vi "dsdll_signal_demo.vi"() -> ()   [LabVIEW 2020, in "dsdll.lvlib"]
doc: "Simple DSDLL demo for measurement of two port system amplitude and phase transfer. \n\nIt generates white noise on mono output and periodically captures waveforms at stereo inputs. \nCaptured wavefroms are displayed and their spectra are calculated. Ratio of their spectra (system frequency response) is filtered and displayed in frequency domain and in nyquist plot."
uses:
  dsdll.lvlib
  dsdll_instance.ctl
  dsdll_device_record.ctl
  dsdll_format.ctl
  dsdll_sample_format.ctl
  dsdll_capture_wave_auto_float32.vi
  dsdll_output_write_auto_float32.vi
panel:
  in  "cut freq":dbl=20000.0 caption="Cut off frequency [Hz]" format="%#_6p"
  out "Nyquist":cluster{dbl[], dbl[]}(graph)
  in  "capt n":u16(ring)=512 caption="Capture samples" items=["64"=64, "128"=128, "256"=256, "512"=512, "1024"=1024, "2048"=2048, "4096"=4096]
  in  "srate":u32=48000 caption="Sample rate [Hz]"
  out "Waveforms":cluster{"fscale":dbl[], dbl[]}[](graph)
  out "A":cdb[](array[numeric])
  out "Transfer":cluster{"fscale":dbl[], dbl[]}[](graph)
  in  "refresh":i32=10 caption="Refresh [ms]" min=0
  in  "btn clr avg":bool
  in  "avg n":u32=5 caption="Averages" min=1
  in  "gen N":i32=7919 caption="Noise generator period"
  in  "btn close":bool
  in  "btn open":bool
  in  "btn exit":bool
  in  "devs capt":u16(ring) caption="Capture devices"
  in  "devs out":u16(ring) caption="Output devices"
  in  "btn enum":bool
  out "error out":errorcluster caption="Error out"
  out "dsdll":T1
  # "DSDLL: Frequency response demo"
  # "Sound card connection:"
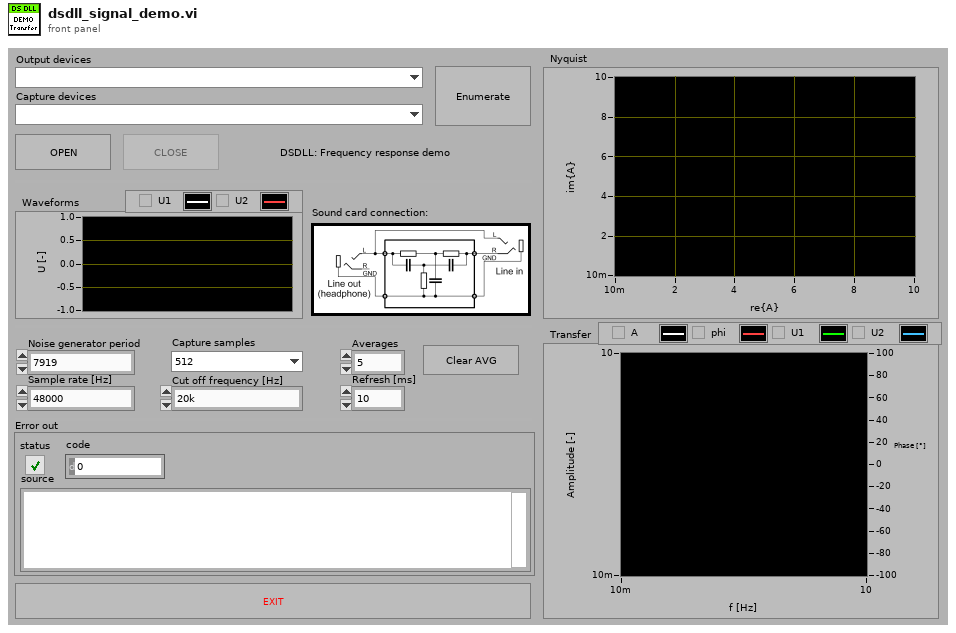
[diagram p1: front panel]
types:
  T1 = typedef "dsdll.lvlib/dsdll_instance.ctl" = cluster{"dsdll path":path, "dsdll handle":u8[], "output devices":T2[], "capture devices":T2[]}
  T2 = typedef "dsdll.lvlib/dsdll_device_record.ctl" = cluster{"guid":u8[], "name":string}
  T3 = typedef "dsdll.lvlib/dsdll_format.ctl" = cluster{"sample rate [Hz]":u32, "out channels":u16, "inp channels":u16, "format":T4}
  T4 = typedef "dsdll.lvlib/dsdll_sample_format.ctl" = enum16{"IEEE float 32", "PCM 16 bit"}
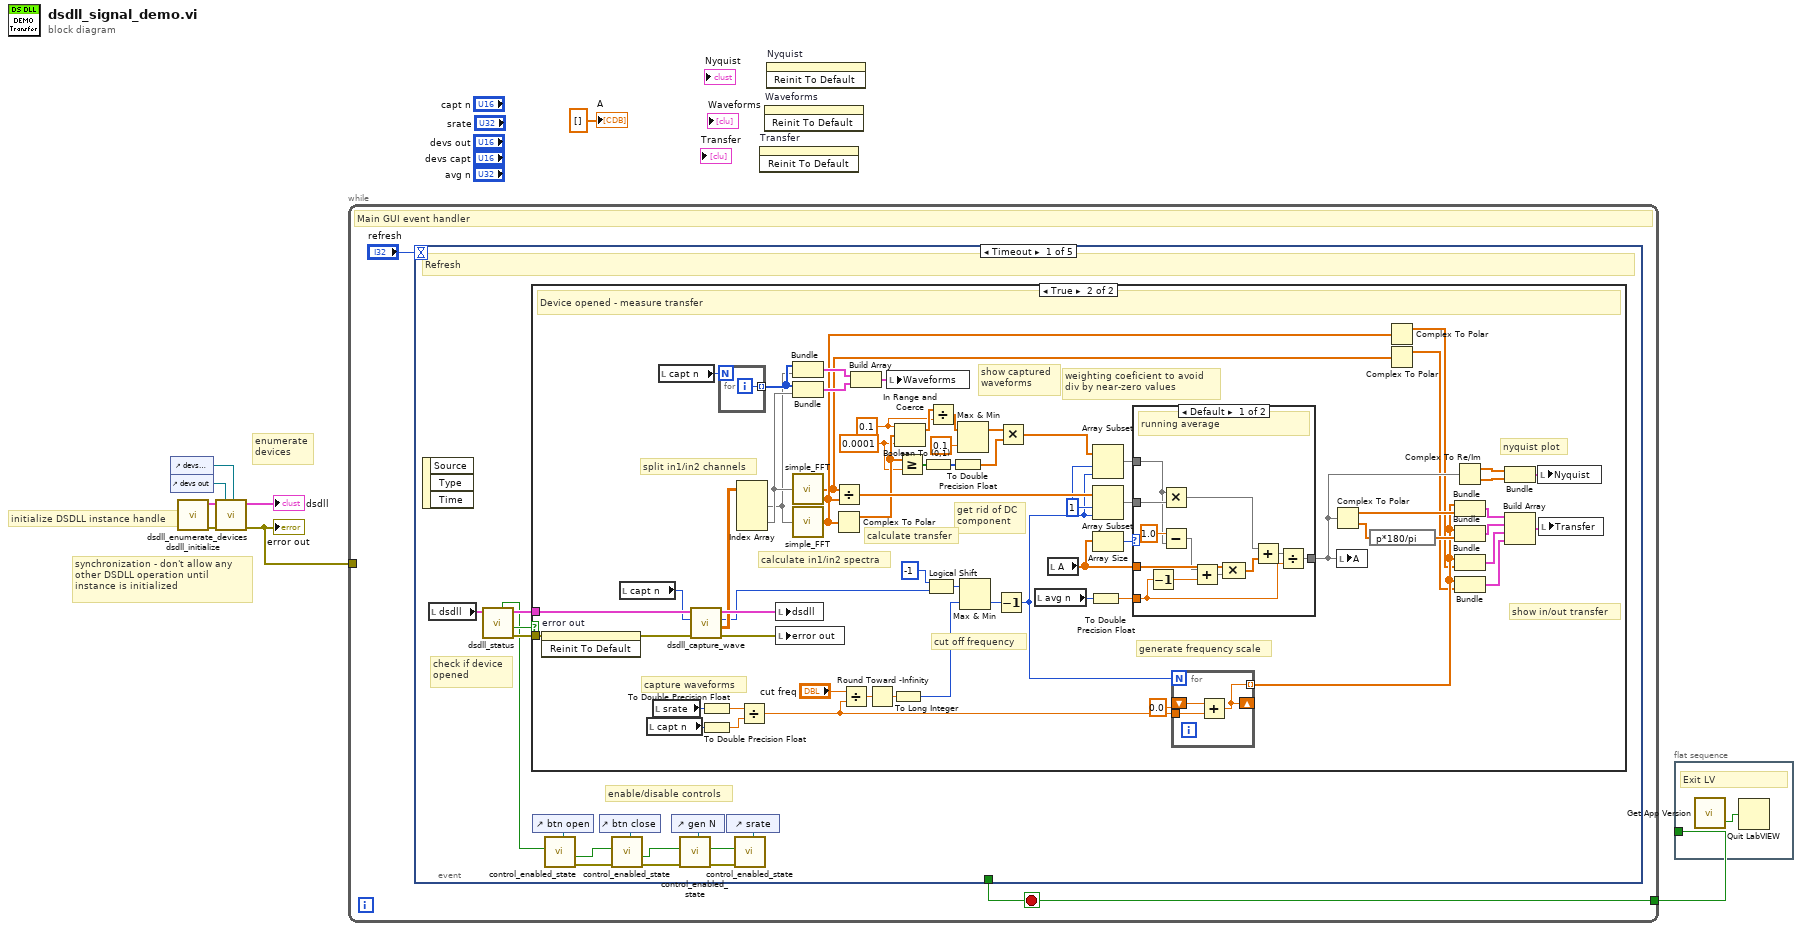
[diagram p0: block diagram]
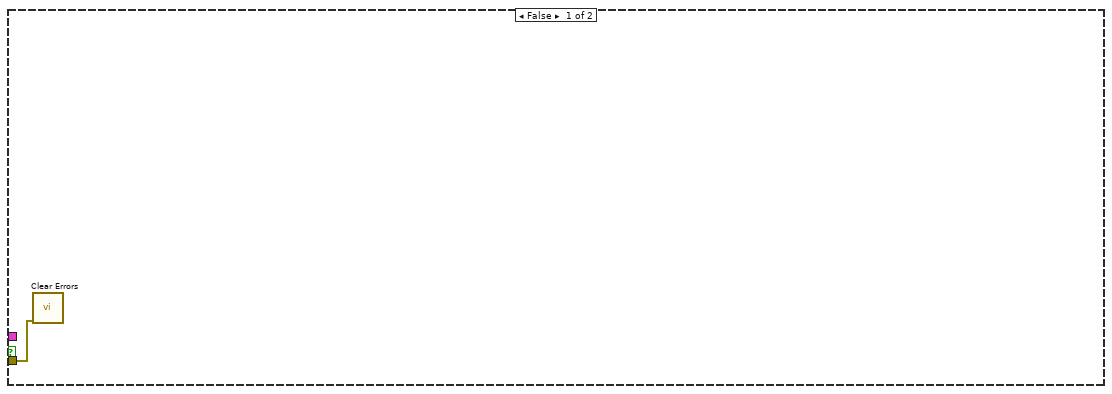
[diagram p2: hidden frame]
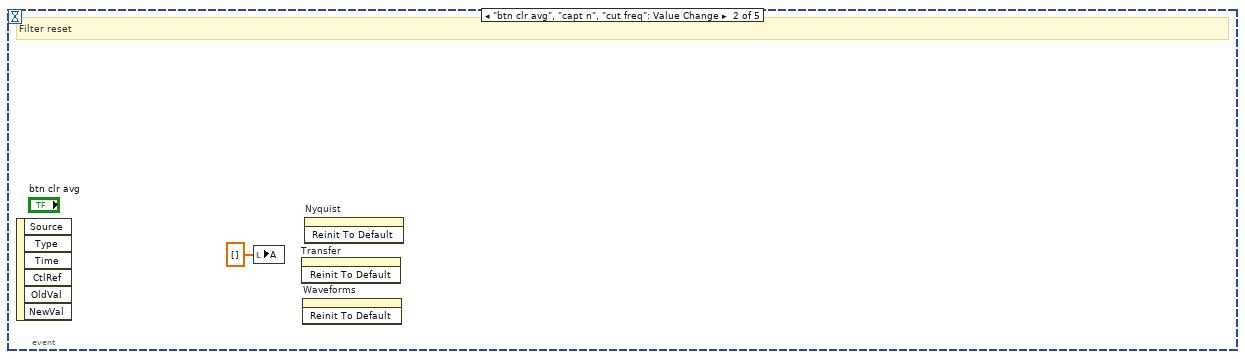
[diagram p4: hidden frame]
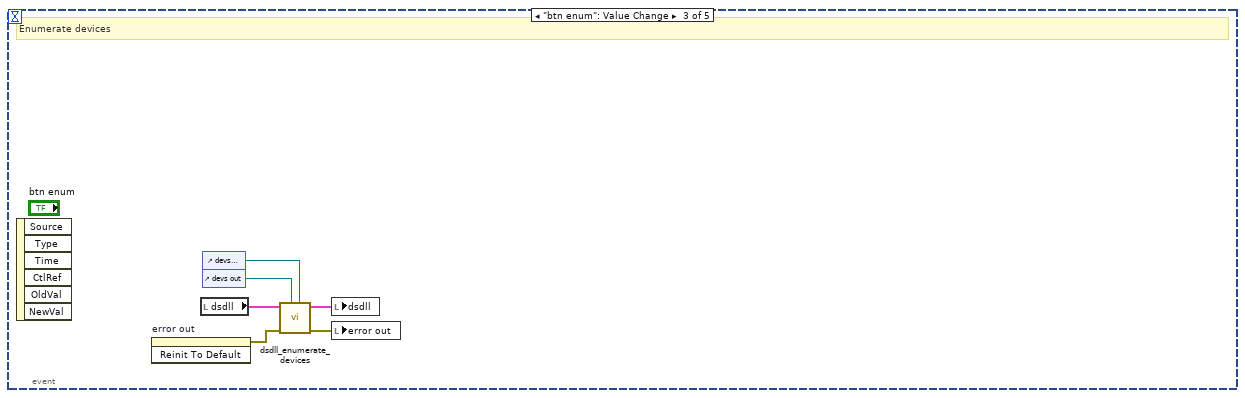
[diagram p5: hidden frame]
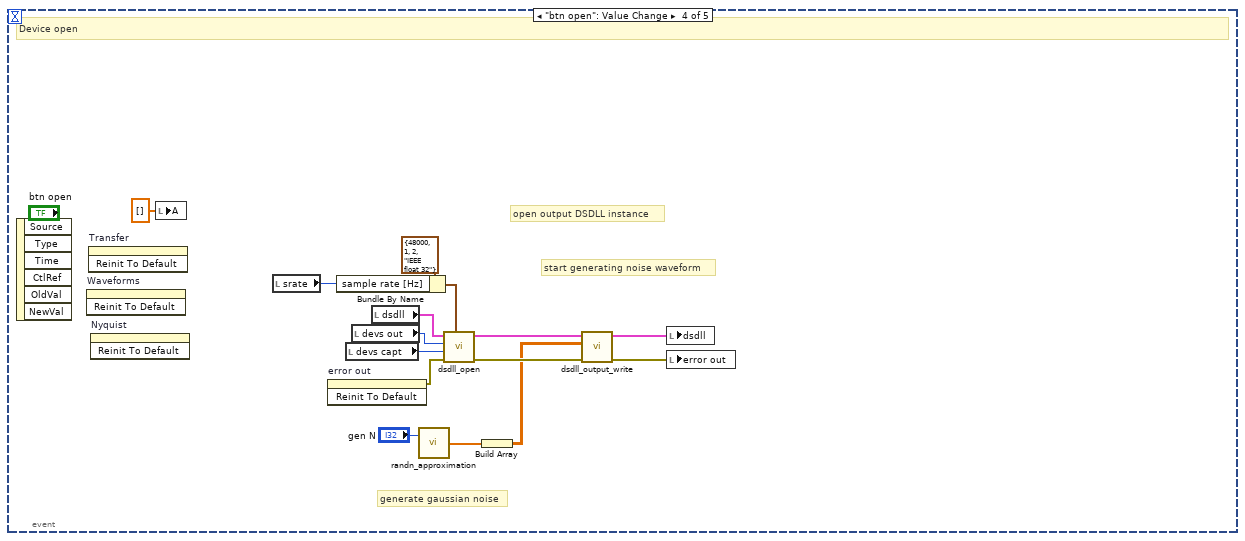
[diagram p6: hidden frame]
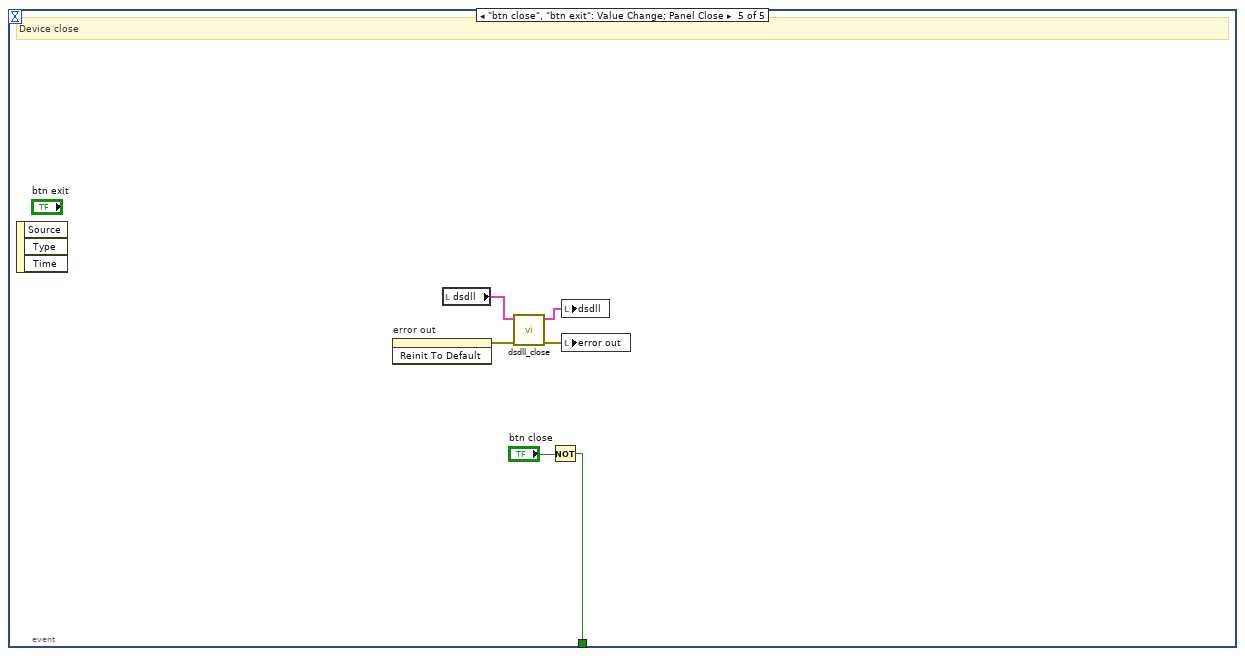
[diagram p7: hidden frame]
diagram:
  # "enumerate\ndevices"
  # "synchronization - don't allow any\nother DSDLL operation until\ninstance is initialized"
  # "initialize DSDLL instance handle"
  n1 = control-ref of="devs capt"() -> (w4:refnum<vi>)
  n2 = control-ref of="devs out"() -> (w5:refnum<vi>)
  n3 = call "dsdll_initialize.vi"() -> ("error out"=w8:errorcluster, "dsdll instance out"=w7:T1)  [unwired: 10 in]
  n4 = call "dsdll_enumerate_devices.vi"("capture devices ring ref"=w4, "output devices ring ref"=w5, "error in"=w8, "dsdll instance in"=w7) -> ("error out"=w2:errorcluster, "dsdll instance out"=→"dsdll":T1)  [unwired: 4 in, 2 out]
  "error out" <- w2
  n5 = while {
    tunnel: [w10] -> w3
    tunnel: w2 -> [_]
    stop <- w10 stop-if-true
    # "Main GUI event handler"
    n6 = event shown="[0] Timeout" {
      selector: _ -> [_ _ _ _ _]
      dyn-events: _ -> [_ _ _ _ _]
      timeout: "refresh" -> [_ _ _ _ _]
      tunnel: [_ _ _ _ w131] -> w10
      event Timeout {
        # "check if device\nopened"
        # "enable/disable controls"
        # "Refresh"
        n7 = event-data() -> ()  [unwired: 1 in, 3 out]
        n8 = local read "dsdll"() -> (w24:T1)
        n9 = call "dsdll_status.vi"("dsdll instance in"=w24) -> ("error out"=w22:errorcluster, "output buffer ok"=w25:bool, "dsdll instance out"=w23:T1, "invalid instance handle"=w19:bool)  [unwired: 5 in, 2 out]
        n10 = case shown="True" w25 {
          tunnel: w23 -> [_ w85]
          tunnel: w22 -> [w26 w69]
          frame False {
            n11 = call <vilib>:"Clear Errors.vi"("error in (no error)"=w26) -> ()  [unwired: 5 in, 2 out]
          }
          frame True {
            w46 = 0.0001
            w34 = 0.1
            w41 = 1 ("index")
            # "weighting coeficient to avoid\ndiv by near-zero values"
            # "split in1/in2 channels"
            # "calculate in1/in2 spectra"
            # "calculate transfer"
            # "get rid of DC\ncomponent"
            # "cut off frequency"
            # "nyquist plot"
            # "show in/out transfer"
            # "capture waveforms"
            # "show captured\nwaveforms"
            # "generate frequency scale"
            # "Device opened - measure transfer"
            n12 = invoke on="error out" class="Clust (strict)" method="Reinit To Default"(error in=w69) -> (error out=w91:errorcluster)  [unwired: 2 in, 2 out]
            n13 = local read "capt n"() -> (w77:u16)
            n14 = local read "capt n"() -> (w54:u16)
            n15 = local read "srate"() -> (w70:u32)
            n16 = local read "capt n"() -> (w72:u16)
            n17 = call-poly "dsdll_capture_wave.vi"("error in"=w91, "samples count in"=w77, "dsdll instance in"=w85) -> ("error out"=w90:errorcluster, "float32 waves"=w88:sgl[][], "samples count out"=w48:u32, "dsdll instance out"=w89:T1)  [unwired: 3 in, 2 out]
            n18 = To Double Precision Float(number=w70) -> (double precision float=w51:dbl)
            n19 = To Double Precision Float(number=w54) -> (double precision float=w53:dbl)
            n20 = for {
              N: w72 -> [_]
              tunnel: [w92] -> w73 mode=indexing
              i -> [w92]
            }
            n21 = Index Array(array=w88) -> (element #1=w49:sgl[], element #2=w50:sgl[])  [unwired: 4 in]
            n22 = Divide(x=w51, y=w53) -> (x/y=w52:dbl)
            n23 = local write "dsdll"(w89) -> ()
            n24 = local write "error out"(w90) -> ()
            n25 = Bundle(w73, "float32 waves"=w49) -> (w74:cluster{i32[], "float32 waves":sgl[]})  [unwired: 1 in]
            n26 = Bundle(w73, "float32 waves"=w50) -> (w75:cluster{i32[], "float32 waves":sgl[]})  [unwired: 1 in]
            n27 = call "simple_FFT.vi"("x(t)"=w50) -> ("X(w)"=w29:cdb[])
            n28 = call "simple_FFT.vi"("x(t)"=w49) -> ("X(w)"=w30:cdb[])
            n29 = Divide(x=w29, y=w30) -> (x/y=w87:cdb[])
            n30 = Complex To Polar(r * e^(i*theta)=w30) -> (r=w47:dbl[])  [unwired: 1 out]
            n31 = Divide(x="cut freq", y=w52) -> (x/y=w59:dbl)
            n32 = Build Array(w74, w75) -> (w71:cluster{i32[], "float32 waves":sgl[]}[])
            n33 = Round Toward -Infinity(1:w59) -> (0:w58:dbl)
            n34 = local write "Waveforms"(w71) -> ()
            n35 = To Long Integer(number=w58) -> (32bit integer=w56:i32)
            n36 = In Range and Coerce(upper limit=w34, x=w47, lower limit=w46) -> (coerced(x)=w36:dbl[])  [unwired: 1 out]
            n37 = Greater Or Equal?(x=w47, y=w46) -> (x >= y?=w45:bool[])
            n38 = Boolean To (0,1)(Boolean=w45) -> (0, 1=w44:i16[])
            n39 = Logical Shift(y=i16 -1, x=w48) -> (x << y=w57:u32)
            n40 = Divide(x=w36, y=w34) -> (x/y=w35:dbl[])
            n41 = To Double Precision Float(number=w44) -> (double precision float=w43:dbl[])
            n42 = Max & Min(x=w35, y=0.1) -> (max(x,y)=w39:dbl[])  [unwired: 1 out]
            n43 = Max & Min(x=w57, y=w56) -> (min(x,y)=w55:u32)  [unwired: 1 out]
            n44 = Decrement(x=w55) -> (x-1=w40:u32)
            n45 = Multiply(x=w39, y=w43) -> (x*y=w42:dbl[])
            n46 = local read "avg n"() -> (w82:u32)
            n47 = local read "A"() -> (w83:cdb[])
            n48 = To Double Precision Float(number=w82) -> (double precision float=w81:dbl)
            n49 = Array Subset(array=w42, index=w41, length=w40) -> (w37:dbl[])
            n50 = Array Subset(array=w87, index=w41, length=w40) -> (w67:cdb[])
            n51 = Array Size(array=w83) -> (size(s)=w84:i32)
            n52 = case shown="Default" w84 {
              tunnel: w83 -> [w107 _]
              tunnel: w81 -> [w103 _]
              tunnel: w67 -> [w102 w108]
              tunnel: [w105 w108] -> w64
              tunnel: w37 -> [w99 _]
              frame Default {
                # "running average"
                n53 = Decrement(x=w103) -> (x-1=w98:dbl)
                n54 = Multiply(x=w99, y=w102) -> (x*y=w101:cdb[])
                n55 = Subtract(x=1.0, y=w99) -> (x-y=w96:dbl[])
                n56 = Add(x=w96, y=w98) -> (x+y=w97:dbl[])
                n57 = Compound Arithmetic op=MULTIPLY(w107, w97) -> (w106:cdb[])
                n58 = Add(x=w101, y=w106) -> (x+y=w104:cdb[])
                n59 = Divide(x=w104, y=w103) -> (x/y=w105:cdb[])
              }
              frame 0 {
                # "filter reset"
              }
            }
            n60 = for {
              N: w40 -> [_]
              tunnel: w52 -> [w95]
              shift-right: [w93] -> _
              shift-left: 0.0 -> [w94]
              tunnel: [w93] -> w31 mode=indexing
              n61 = Add(x=w94, y=w95) -> (x+y=w93:dbl)
            }
            n62 = Complex To Polar(r * e^(i*theta)=w64) -> (r=w63:dbl[], theta=w61:dbl[])
            n63 = local write "A"(w64) -> ()
            n64 = expression code="p*180/pi"(w61) -> (w62:dbl[])
            n65 = Complex To Polar(r * e^(i*theta)=w30) -> (r=w27:dbl[])  [unwired: 1 out]
            n66 = Complex To Polar(r * e^(i*theta)=w29) -> (r=w28:dbl[])  [unwired: 1 out]
            n67 = Complex To Re/Im(x + iy=w64) -> (x=w66:dbl[], y=w65:dbl[])
            n68 = Bundle(w31, w63) -> (w80:cluster{dbl[], dbl[]})  [unwired: 1 in]
            n69 = Bundle(w31, w62) -> (w79:cluster{dbl[], dbl[]})  [unwired: 1 in]
            n70 = Bundle(w31, w27) -> (w33:cluster{dbl[], dbl[]})  [unwired: 1 in]
            n71 = Bundle(w31, w28) -> (w32:cluster{dbl[], dbl[]})  [unwired: 1 in]
            n72 = Bundle(w66, w65) -> (w68:cluster{dbl[], dbl[]})  [unwired: 1 in]
            n73 = Build Array(w80, w79, w33, w32) -> (w78:cluster{dbl[], dbl[]}[])
            n74 = local write "Nyquist"(w68) -> ()
            n75 = local write "Transfer"(w78) -> ()
          }
        }
        n76 = control-ref of="btn open"() -> (w21:refnum<vi>)
        n77 = call "control_enabled_state.vi"("enabled"=w19, "control in"=w21) -> ("error out"=w11:errorcluster, "disabled"=w18:bool)  [unwired: 6 in, 2 out]
        n78 = control-ref of="btn close"() -> (w20:refnum<vi>)
        n79 = call "control_enabled_state.vi"("error in (no error)"=w11, "enabled"=w18, "control in"=w20) -> ("error out"=w12:errorcluster, "disabled"=w16:bool)  [unwired: 5 in, 2 out]
        n80 = control-ref of="gen N"() -> (w17:refnum<vi>)
        n81 = call "control_enabled_state.vi"("error in (no error)"=w12, "enabled"=w16, "control in"=w17) -> ("error out"=w14:errorcluster, "enabled"=w13:bool)  [unwired: 5 in, 2 out]
        n82 = control-ref of="srate"() -> (w15:refnum<vi>)
        n83 = call "control_enabled_state.vi"("error in (no error)"=w14, "enabled"=w13, "control in"=w15) -> ()  [unwired: 5 in, 4 out]
      }
      event "btn clr avg", "capt n", "cut freq": Value Change {
        # "Filter reset"
        n84 = event-data() -> ()  [unwired: 1 in, 6 out]
        n85 = local write "A"(cdb[] [] ("tf")) -> ()
        n86 = invoke on="Transfer" class="XYGraph (strict)" method="Reinit To Default"() -> ()  [unwired: 3 in, 3 out]
        n87 = invoke on="Waveforms" class="XYGraph (strict)" method="Reinit To Default"() -> ()  [unwired: 3 in, 3 out]
        n88 = invoke on="Nyquist" class="XYGraph (strict)" method="Reinit To Default"() -> ()  [unwired: 3 in, 3 out]
      }
      event "btn enum": Value Change {
        # "Enumerate devices"
        n89 = event-data() -> ()  [unwired: 1 in, 6 out]
        n90 = invoke on="error out" class="Clust (strict)" method="Reinit To Default"() -> (error out=w110:errorcluster)  [unwired: 3 in, 2 out]
        n91 = local read "dsdll"() -> (w115:T1)
        n92 = control-ref of="devs capt"() -> (w112:refnum<vi>)
        n93 = control-ref of="devs out"() -> (w113:refnum<vi>)
        n94 = call "dsdll_enumerate_devices.vi"("capture devices ring ref"=w112, "output devices ring ref"=w113, "error in"=w110, "dsdll instance in"=w115) -> ("error out"=w114:errorcluster, "dsdll instance out"=w111:T1)  [unwired: 4 in, 2 out]
        n95 = local write "dsdll"(w111) -> ()
        n96 = local write "error out"(w114) -> ()
      }
      event "btn open": Value Change {
        # "start generating noise waveform"
        # "open output DSDLL instance"
        # "generate gaussian noise"
        # "Device open"
        n97 = event-data() -> ()  [unwired: 1 in, 6 out]
        n98 = invoke on="Waveforms" class="XYGraph (strict)" method="Reinit To Default"() -> ()  [unwired: 3 in, 3 out]
        n99 = invoke on="Transfer" class="XYGraph (strict)" method="Reinit To Default"() -> ()  [unwired: 3 in, 3 out]
        n100 = invoke on="Nyquist" class="XYGraph (strict)" method="Reinit To Default"() -> ()  [unwired: 3 in, 3 out]
        n101 = local write "A"(cdb[] [] ("tf")) -> ()
        n102 = local read "srate"() -> (w118:u32)
        n103 = invoke on="error out" class="Clust (strict)" method="Reinit To Default"() -> (error out=w127:errorcluster)  [unwired: 3 in, 2 out]
        n104 = Bundle By Name(cluster=T3 {"sample rate [Hz]"=48000, "out channels"=1, "inp channels"=2, "format"=enum."IEEE float 32"} ("format"), "sample rate [Hz]"=w118) -> (w116:T3)
        n105 = local read "devs capt"() -> (w129:u16)
        n106 = local read "devs out"() -> (w128:u16)
        n107 = local read "dsdll"() -> (w130:T1)
        n108 = call "randn_approximation.vi"("N"="gen N") -> ("randn() vector"=w121:dbl[])  [unwired: 1 in]
        n109 = call "dsdll_open.vi"("format"=w116, "error in"=w127, "capture device id"=w129, "output device id"=w128, "dsdll instance in"=w130) -> ("error out"=w125:errorcluster, "dsdll instance out"=w122:T1)  [unwired: 5 in]
        n110 = Build Array(w121) -> (w120:dbl[][])
        n111 = call-poly "dsdll_output_write.vi"("error in"=w125, "float32 samples"=w120, "dsdll instance in"=w122) -> ("error out"=w124:errorcluster, "dsdll instance out"=w123:T1)  [unwired: 7 in]
        n112 = local write "dsdll"(w123) -> ()
        n113 = local write "error out"(w124) -> ()
      }
      event "btn close", "btn exit": Value Change; Panel Close {
        # "Device close"
        n114 = event-data() -> ()  [unwired: 1 in, 3 out]
        n115 = invoke on="error out" class="Clust (strict)" method="Reinit To Default"() -> (error out=w133:errorcluster)  [unwired: 3 in, 2 out]
        n116 = local read "dsdll"() -> (w134:T1)
        n117 = call "dsdll_close.vi"("error in"=w133, "dsdll instance in"=w134) -> ("error out"=w136:errorcluster, "dsdll instance out"=w135:T1)  [unwired: 8 in]
        n118 = Not(x="btn close") -> (.not. x?=w131:bool)
        n119 = local write "dsdll"(w135) -> ()
        n120 = local write "error out"(w136) -> ()
      }
    }
  }
  n121 = invoke on="Transfer" class="XYGraph (strict)" method="Reinit To Default"() -> ()  [unwired: 3 in, 3 out]
  n122 = invoke on="Waveforms" class="XYGraph (strict)" method="Reinit To Default"() -> ()  [unwired: 3 in, 3 out]
  n123 = invoke on="Nyquist" class="XYGraph (strict)" method="Reinit To Default"() -> ()  [unwired: 3 in, 3 out]
  n124 = flat-sequence {
    tunnel: w3 -> [_]
    frame #0 {
      # "Exit LV"
      n125 = call "Get App Version.vi"() -> ("runtime"=w137:bool)  [unwired: 1 out]
      n126 = Quit LabVIEW(quit? (T)=w137) -> ()
    }
  }
  "A" <- cdb[] [] ("tf")
